vi "Close Dictionary.vi"(8 "error in (no error)":errorcluster, 11 "Control Experiment in":refnum<class "Control Experiment.lvclass">) -> (0 "error out":errorcluster, 3 "Control Experiment out":refnum<class "Control Experiment.lvclass">)   [LabVIEW 2019, in "Control Experiment.lvclass"]
uses:
  Control Experiment.lvclass
  <userlib>/_OpenG.lib/dictionary/dictionary.llb/Dictionary Object RefNum__ogtk.ctl
  <userlib>/_OpenG.lib/dictionary/dictionary.llb/Dictionary Object RefNum - Enum__ogtk.ctl
  Control Experiment.lvclass/Control Experiment.ctl
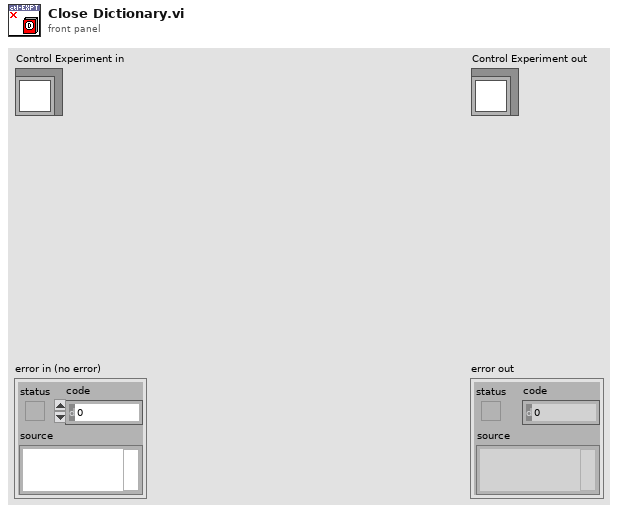
[diagram p1: front panel]
types:
  T1 = typedef "Dictionary Object RefNum__ogtk.ctl" = refnum<k1>
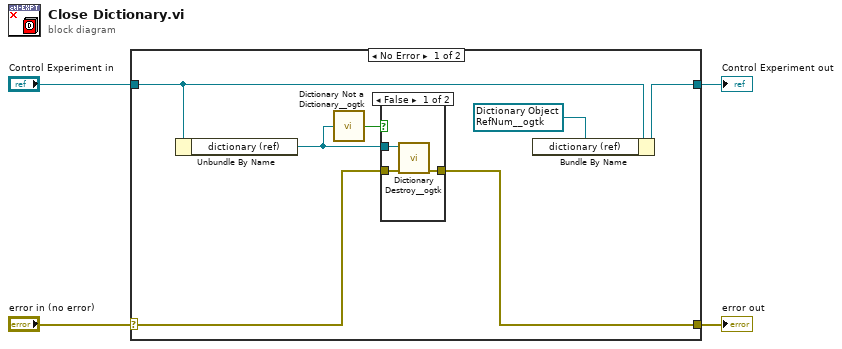
[diagram p0: block diagram]
diagram:
  n1 = case shown="No Error" "error in (no error)" {
    selector: "error in (no error)" -> [w8 w16]
    tunnel: [w5 w16] -> w3
    tunnel: [w11 w17] -> w1
    tunnel: "Control Experiment in" -> [w10 w17]
    frame No Error {
      w6 = T1 refnum items=["Dictionary"] ("Experiment.dictionary")
      n2 = Unbundle By Name(w10) -> ("dictionary (ref)"=w7:T1)
      n3 = call <userlib>:"Dictionary Not a Dictionary__ogtk.vi"("dictionary"=w7) -> ("not a dictionary?"=w9:bool)
      n4 = case shown="False" w9 {
        tunnel: w7 -> [w13 _]
        tunnel: w8 -> [w14 w15]
        tunnel: [w12 w15] -> w5
        frame False {
          n5 = call <userlib>:"Dictionary Destroy__ogtk.vi"("error in (no error)"=w14, "dictionary"=w13) -> ("error out"=w12:errorcluster)  [unwired: 9 in]
        }
        frame True {
        }
      }
      n6 = Bundle By Name(cluster=w10, "dictionary (ref)"=w6) -> (w11:refnum<class "Control Experiment.lvclass">)
    }
    frame Error {
    }
  }
  "error out" <- w3
  "Control Experiment out" <- w1
